vi "DashboardCore.vi"(11 "Plugin Info":T1) -> ()   [LabVIEW 2015]
uses:
  CorePluginInfo.ctl
  CoreDashGlobal.vi
panel:
  in  "TCP":refnum<k5>
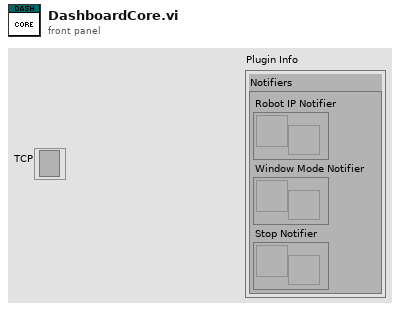
[diagram p1: front panel]
types:
  T1 = typedef "CorePluginInfo.ctl" = cluster{"Notifiers":cluster{"Robot IP Notifier":refnum<notifier>, "Window Mode Notifier":refnum<notifier>, "Stop Notifier":refnum<notifier>}}
  T2 = cluster{"Error Strings":string, "Disable Counts":cluster{u16, u16}, "Rail Faults":cluster{u16, u16, u16}, "Robot IP":string, "DB Mode":u8, "Event Info":cluster{"Name":string, "Type":u8, "Number":u16, "Replay":u8}, "Camera Addr":string}
  T3 = cluster{"Storage":cluster{"Disk Free":u64, "RAM Block":u32, "RAM free":u32}, "CPU Utilization":cluster{"CPU % ISR":sgl, "CPU % Time Crit":sgl, "CPU % Timed Str":sgl, "CPU % High":sgl, "CPU % Above":sgl, "CPU % Normal":sgl, "CPU % Low":sgl}, "CAN":cluster{"% Bus Utilization":sgl, "Bus Off Cnt":u32, "TX_FIFO Full Cnt":u32, "Receive Error Cnt":u8, "Transmit Error Cnt":u8}, "HID":cluster{"HID Outputs":u32, "Rumble Low":u16, "Rumble High":u16}[]}
  T4 = cluster{"Status bits":cluster{"Test Mode":bool, "Autonomous":bool, "Enabled":bool, "Code Start":bool, "Brownout":bool, "Reserved 2":bool, "Reserved 3":bool, "E-Stop":bool}, "Code Trace":cluster{"Disabled":bool, "TeleOp":bool, "Auto":bool, "Test":bool}, "Controller Type":enum16{"unknown", "cRIO", "roboRio"}, "Code?":enum16{"unknown", "noCode", "code"}, "Battery V":dbl}
  T5 = cluster{"Control Bits":cluster{"TestMode":bool, "Autonomous":bool, "Enabled":bool, "FMS Present":bool, bool, bool, bool, "E-Stop":bool}, "Team Station ":u8, "Countdown":sgl, "Joystick Values":cluster{"Axes":dbl[], "Buttons":bool[], "POVs":i16[]}[]}
  T6 = enum8{"Tele-Op Disabled", "Tele-Op Enabled", "Auto Disabled", "Auto Enabled", "Test Disabled", "Test Enabled", "Disconnected", "No Code", "E-Stop"}
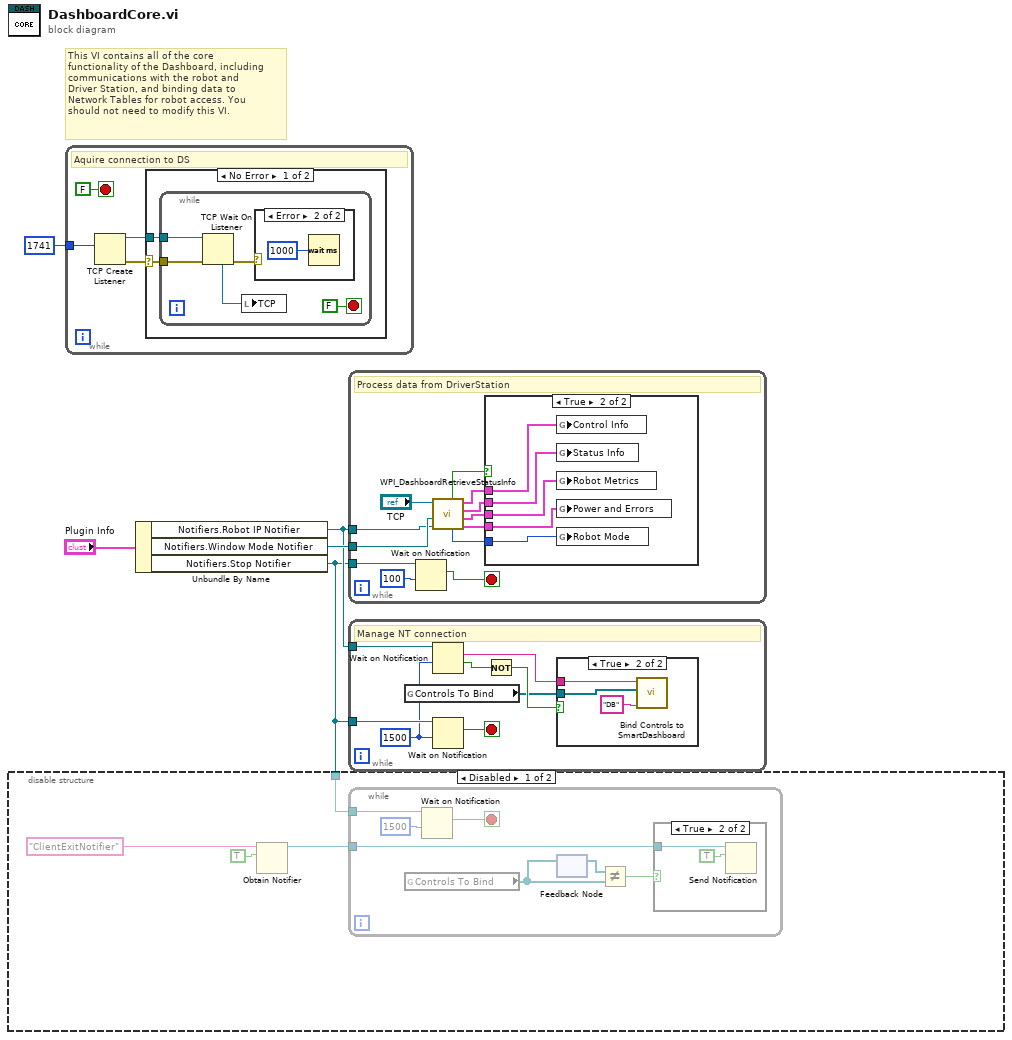
[diagram p0: block diagram]
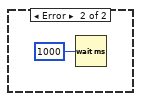
[diagram p6: hidden frame]
diagram:
  # "This VI contains all of the core\nfunctionality of the Dashboard, including\ncommunications with the robot and\nDriver Station, and binding data to \nNetwork Tables for robot access. You\nshould not need to modify this VI."
  n1 = while {
    tunnel: u16 1741 ("timeout ms (25000)") -> [w7]
    stop <- FALSE stop-if-true
    # "Aquire connection to DS"
    n2 = TCP Create Listener(10:w7) -> (0:w6:errorcluster, 3:w8:refnum<k5>)  [unwired: 4 in, 1 out]
    n3 = case shown="No Error" w6 {
      selector: w6 -> [w10 _]
      tunnel: w8 -> [w11 _]
      frame No Error {
        n4 = while {
          tunnel: w11 -> [w15]
          tunnel: w10 -> [w14]
          stop <- FALSE stop-if-true
          n5 = TCP Wait On Listener(8:w14, 11:w15) -> (0:w16:errorcluster, 4:w12:refnum<k5>)  [unwired: 2 in, 3 out]
          n6 = local write "TCP"(w12) -> ()
          n7 = case shown="Error" w16 {
            frame No Error {
            }
            frame Error {
              n8 = Wait (ms)(milliseconds to wait=u32 1000) -> ()  [unwired: 1 out]
            }
          }
        }
      }
      frame Error {
        n9 = Wait (ms)(milliseconds to wait=u32 1000) -> ()  [unwired: 1 out]
      }
    }
  }
  n10 = Unbundle By Name("Plugin Info") -> ("Notifiers.Robot IP Notifier"=w2:refnum<notifier>, "Notifiers.Window Mode Notifier"=w3:refnum<notifier>, "Notifiers.Stop Notifier"=w1:refnum<notifier>)
  n11 = disable-structure shown="Disabled" {
    disable-tunnel: w1 -> [w19 _]
    frame Disabled {
      n12 = Obtain Notifier(name (unnamed)="ClientExitNotifier", notification data type=TRUE) -> (notifier out=w20:refnum<notifier>)  [unwired: 2 in, 2 out]
      n13 = while {
        tunnel: w20 -> [w26]
        tunnel: w19 -> [w23]
        stop <- w24 stop-if-true
        n14 = global read "CoreDashGlobal.vi" "Controls To Bind"() -> (w29:refnum<vi>[])
        n15 = Wait on Notification(notifier=w23, timeout in ms (-1)=1500) -> (notification=w24:bool)  [unwired: 2 in, 3 out]
        n16 = feedback #1() -> (w28:refnum<vi>[])  [unwired: 1 in]
        n17 = feedback-in #1(w29) -> ()
        n18 = Not Equal?(x=w28, y=w29) -> (x != y?=w27:bool)
        n19 = case shown="True" w27 {
          tunnel: w26 -> [_ w31]
          frame False {
          }
          frame True {
            n20 = Send Notification(notification=TRUE, notifier=w31) -> ()  [unwired: 1 in, 2 out]
          }
        }
      }
    }
    frame Enabled {
    }
  }
  n21 = while {
    tunnel: w3 -> [w42]
    tunnel: w2 -> [w41]
    tunnel: w1 -> [w33]
    stop <- w32 stop-if-true
    # "Process data from DriverStation"
    n22 = Wait on Notification(notifier=w33, timeout in ms (-1)=100) -> (notification=w32:bool)  [unwired: 2 in, 3 out]
    n23 = call <vilib>:"WPI_DashboardRetrieveStatusInfo.vi"("Binding Refnum"=w41, "Window Mode Notifier"=w42, "TCP Cnx"="TCP") -> ("Power and Errors"=w37:T2, "Robot Metrics"=w38:T3, "Status Info"=w39:T4, "Control Info"=w40:T5, "Robot Mode"=w36:T6, "Process?"=w35:bool)  [unwired: 3 in]
    n24 = case shown="True" w35 {
      tunnel: w40 -> [_ w48]
      tunnel: w39 -> [_ w47]
      tunnel: w38 -> [_ w46]
      tunnel: w37 -> [_ w45]
      tunnel: w36 -> [_ w44]
      frame False {
      }
      frame True {
        n25 = global write "CoreDashGlobal.vi" "Control Info"(w48) -> ()
        n26 = global write "CoreDashGlobal.vi" "Status Info"(w47) -> ()
        n27 = global write "CoreDashGlobal.vi" "Robot Metrics"(w46) -> ()
        n28 = global write "CoreDashGlobal.vi" "Power and Errors"(w45) -> ()
        n29 = global write "CoreDashGlobal.vi" "Robot Mode"(w44) -> ()
      }
    }
  }
  n30 = while {
    tunnel: w2 -> [w56]
    tunnel: w1 -> [w51]
    stop <- w49 stop-if-true
    w50 = 1500 ("timeout in ms (-1)")
    # "Manage NT connection"
    n31 = global read "CoreDashGlobal.vi" "Controls To Bind"() -> (w52:refnum<vi>[])
    n32 = Wait on Notification(notifier=w56, timeout in ms (-1)=w50) -> (notification=w53:string, timed out?=w55:bool)  [unwired: 2 in, 2 out]
    n33 = Wait on Notification(notifier=w51, timeout in ms (-1)=w50) -> (notification=w49:bool)  [unwired: 2 in, 3 out]
    n34 = Not(x=w55) -> (.not. x?=w54:bool)
    n35 = case shown="True" w54 {
      tunnel: w53 -> [_ w59]
      tunnel: w52 -> [_ w58]
      frame False {
      }
      frame True {
        n36 = call <vilib>:"Bind Controls to SmartDashboard.vi"("Client Name"="DB", "Bound Control Refs"=w58, "Server IP Address"=w59) -> ()  [unwired: 9 in]
      }
    }
  }
